vi "VI Tree.vi"   [LabVIEW 2012, in "Stanford Research 830.lvlib"]
doc: "This is the instrument driver for the Stanford Research 810/830. The VI Tree displays all the user-callable VIs of the instrument driver in an organized table."
uses:
  <instrlib>/Stanford Research 830/Stanford Research 830.lvlib
  <instrlib>/Stanford Research 830/Public/Data/Read (Multiple Points).vi
  <instrlib>/Stanford Research 830/Public/Data/Read (All Parameters).vi
  <instrlib>/Stanford Research 830/Public/Data/Read (1 Parameter).vi
panel:
  # "(c) 2006 National Instruments.  ALL RIGHTS RESERVED."
  # "SEE DIAGRAM\nFOR VI TREE."
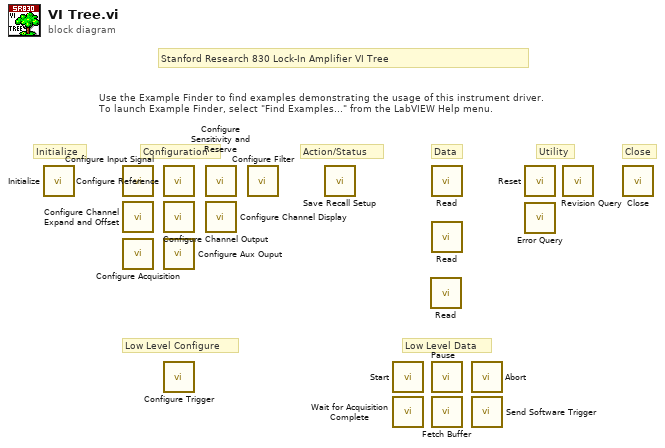
[diagram p0: block diagram]
diagram:
  # "Low Level Configure"
  # "Close"
  # "Utility"
  # "Data"
  # "Action/Status"
  # "Configuration"
  # "Initialize"
  # "Low Level Data"
  # "Stanford Research 830 Lock-In Amplifier VI Tree"
  # "Use the Example Finder to find examples demonstrating the usage of this instrument driver.\nTo launch Example Finder, select \"Find Examples...\" from the LabVIEW Help menu."
  n1 = call <instrlib>:"Initialize.vi"() -> ()  [unwired: 10 in, 2 out]
  n2 = call <instrlib>:"Configure Input Signal.vi"() -> ()  [unwired: 10 in, 2 out]
  n3 = call <instrlib>:"Configure Channel Expand and Offset.vi"() -> ()  [unwired: 10 in, 2 out]
  n4 = call <instrlib>:"Configure Acquisition.vi"() -> ()  [unwired: 10 in, 2 out]
  n5 = call <instrlib>:"Configure Reference.vi"() -> ()  [unwired: 14 in, 2 out]
  n6 = call <instrlib>:"Configure Channel Output.vi"() -> ()  [unwired: 10 in, 2 out]
  n7 = call <instrlib>:"Configure Aux Ouput.vi"() -> ()  [unwired: 10 in, 2 out]
  n8 = call <instrlib>:"Configure Trigger.vi"() -> ()  [unwired: 10 in, 2 out]
  n9 = call <instrlib>:"Configure Sensitivity and Reserve.vi"() -> ()  [unwired: 10 in, 2 out]
  n10 = call <instrlib>:"Configure Channel Display.vi"() -> ()  [unwired: 10 in, 2 out]
  n11 = call <instrlib>:"Configure Filter.vi"() -> ()  [unwired: 10 in, 2 out]
  n12 = call <instrlib>:"Save Recall Setup.vi"() -> ()  [unwired: 10 in, 2 out]
  n13 = call <instrlib>:"Start.vi"() -> ()  [unwired: 10 in, 2 out]
  n14 = call <instrlib>:"Wait for Acquisition Complete.vi"() -> ()  [unwired: 10 in, 2 out]
  n15 = call-poly <instrlib>:"Read.vi"() -> ()  [unwired: 9 in, 3 out]
  n16 = call-poly <instrlib>:"Read.vi"() -> ()  [unwired: 9 in, 3 out]
  n17 = call-poly <instrlib>:"Read.vi"() -> ()  [unwired: 9 in, 3 out]
  n18 = call <instrlib>:"Pause.vi"() -> ()  [unwired: 10 in, 2 out]
  n19 = call <instrlib>:"Fetch Buffer.vi"() -> ()  [unwired: 9 in, 3 out]
  n20 = call <instrlib>:"Abort.vi"() -> ()  [unwired: 10 in, 2 out]
  n21 = call <instrlib>:"Send Software Trigger.vi"() -> ()  [unwired: 10 in, 2 out]
  n22 = call <instrlib>:"Reset.vi"() -> ()  [unwired: 10 in, 2 out]
  n23 = call <instrlib>:"Error Query.vi"() -> ()  [unwired: 9 in, 3 out]
  n24 = call <instrlib>:"Revision Query.vi"() -> ()  [unwired: 8 in, 4 out]
  n25 = call <instrlib>:"Close.vi"() -> ()  [unwired: 11 in, 1 out]
